vi "sigmoid_backward.vi"(1 "Z":dbl[][](array[numeric]), 2 "dA":dbl[][](array[numeric])) -> (0 "dZ":dbl[][](array[numeric]))   [LabVIEW 2020]
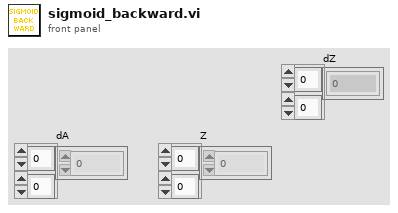
[diagram p1: front panel]
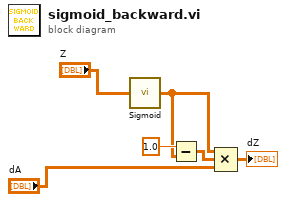
[diagram p0: block diagram]
diagram:
  n1 = call "Sigmoid.vi"("Z"="Z") -> ("Sigmoid(Z)"=w4:dbl[][])  [unwired: 2 in]
  n2 = Subtract(x=1.0, y=w4) -> (x-y=w3:dbl[][])
  n3 = Compound Arithmetic op=MULTIPLY(w4, w3, "dA") -> (→"dZ":dbl[][])
